vi "FGV Exit.vi"(7 "CMD":T1(ring), 8 "error in (no error)":errorcluster, 11 "Exit In":bool) -> (0 "error out":errorcluster, 3 "Exit":bool)   [LabVIEW 2021]
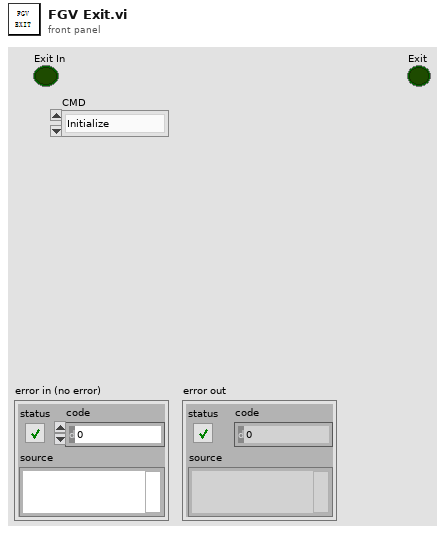
[diagram p1: front panel]
types:
  T1 = enum16{"Initialize", "Read", "Write", "UnInitialize"}
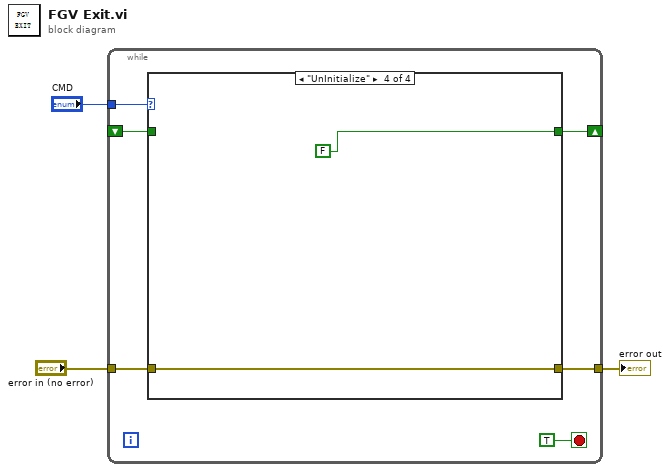
[diagram p0: block diagram]
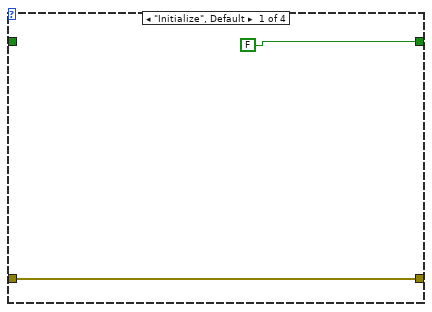
[diagram p2: hidden frame]
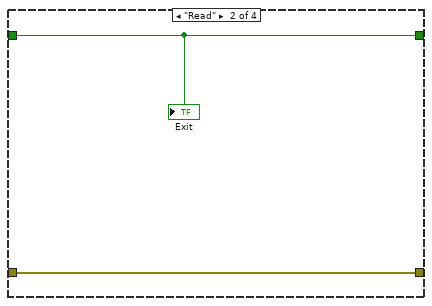
[diagram p3: hidden frame]
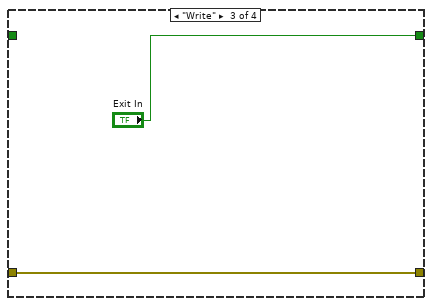
[diagram p4: hidden frame]
diagram:
  n1 = while {
    tunnel: "CMD" -> [w8]
    shift-right: [w6] -> _
    shift-left: _ -> [w7]
    tunnel: "error in (no error)" -> [w5]
    tunnel: [w4] -> w3
    stop <- TRUE stop-if-true
    n2 = case shown="\"UnInitialize\"" w8 {
      tunnel: w7 -> [_ w13 _ _]
      tunnel: [FALSE w13 "Exit In" FALSE ("Exit In")] -> w6
      tunnel: w5 -> [w11 w12 w15 w17]
      tunnel: [w11 w12 w15 w17] -> w4
      frame "Initialize", Default {
      }
      frame "Read" {
        "Exit" <- w13
      }
      frame "Write" {
      }
      frame "UnInitialize" {
      }
    }
  }
  "error out" <- w3
